vi "pmu_Phasor Scale CFG-3.vi"(8 "phasors in":csg[](array[numeric]), 9 "phasor angle offsets [rad]":sgl[](array[numeric]), 10 "phasor scale factors":sgl[](array[numeric]), 11 "format":u16) -> (2 "phasor out of range":bool, 3 "phasor byte array":u8[](array[numeric]))   [LabVIEW 2014, in "NI_EP_PMU.lvlib"]
uses:
  <vilib>/addons/Electrical Power/PMU/NI_EP_PMU.lvlib
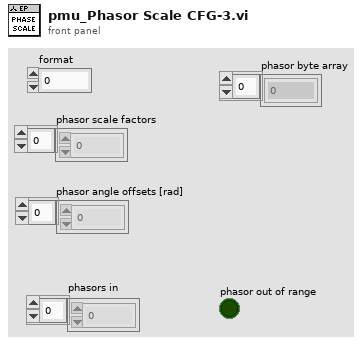
[diagram p1: front panel]
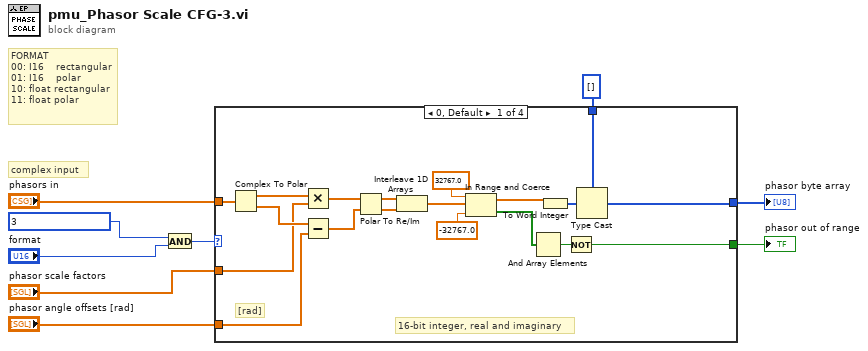
[diagram p0: block diagram]
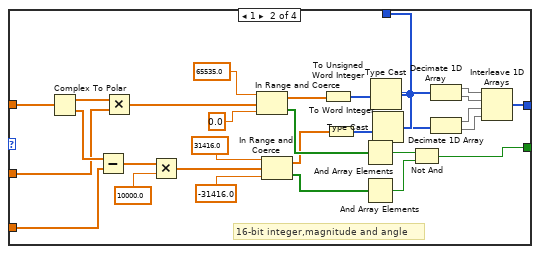
[diagram p2: hidden frame]
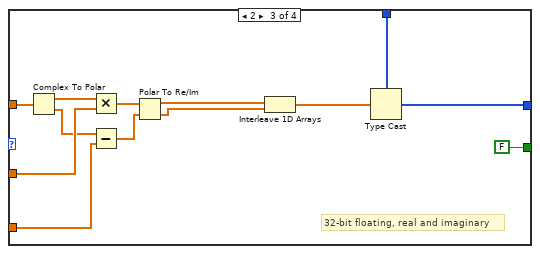
[diagram p3: hidden frame]
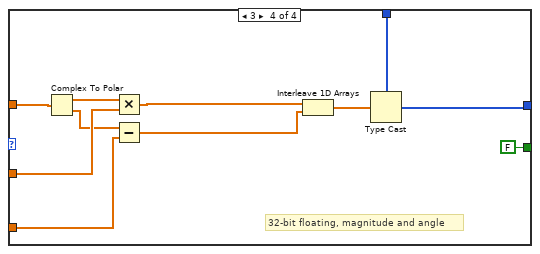
[diagram p4: hidden frame]
diagram:
  # "FORMAT\n00: I16    rectangular\n01: I16    polar\n10: float rectangular\n11: float polar"
  # "complex input"
  n1 = And(x=u16 3, y="format") -> (x .and. y?=w7:u16)
  n2 = case shown="0, Default" w7 {
    tunnel: "phasors in" -> [w23 w58 w67 w78]
    tunnel: u8[] [] ("appended array") -> [w24 w43 w70 w81]
    tunnel: [w28 w36 w69 w80] -> w4
    tunnel: [w25 w35 FALSE FALSE] -> w3
    tunnel: "phasor scale factors" -> [w12 w30 w65 w76]
    tunnel: "phasor angle offsets [rad]" -> [w11 w29 w63 w74]
    frame 0, Default {
      # "[rad]"
      # "16-bit integer, real and imaginary"
      n3 = Complex To Polar(r * e^(i*theta)=w23) -> (r=w22:sgl[], theta=w21:sgl[])
      n4 = Multiply(x=w22, y=w12) -> (x*y=w20:sgl[])
      n5 = Subtract(x=w21, y=w11) -> (x-y=w10:sgl[])
      n6 = Polar To Re/Im(2:w10, 3:w20) -> (0:w18:sgl[], 1:w19:sgl[])
      n7 = Interleave 1D Arrays(w19, w18) -> (w15:sgl[])
      n8 = In Range and Coerce(upper limit=sgl 32767.0, x=w15, lower limit=sgl -32767.0) -> (coerced(x)=w14:sgl[], In Range?=w13:bool[])
      n9 = And Array Elements(Boolean array=w13) -> (logical AND=w26:bool)
      n10 = To Word Integer(number=w14) -> (16bit integer=w27:i16[])
      n11 = Not(x=w26) -> (.not. x?=w25:bool)
      n12 = Type Cast(type=w24, x=w27) -> (*(type *) &x=w28:u8[])
    }
    frame 1 {
      # "16-bit integer,magnitude and angle"
      n13 = Complex To Polar(r * e^(i*theta)=w58) -> (r=w57:sgl[], theta=w34:sgl[])
      n14 = Subtract(x=w34, y=w29) -> (x-y=w32:sgl[])
      n15 = Multiply(x=w57, y=w30) -> (x*y=w56:sgl[])
      n16 = Multiply(x=w32, y=sgl 10000.0) -> (x*y=w33:sgl[])
      n17 = In Range and Coerce(upper limit=sgl 65535.0, x=w56, lower limit=sgl 0.0) -> (coerced(x)=w48:sgl[], In Range?=w51:bool[])
      n18 = In Range and Coerce(upper limit=sgl 31416.0, x=w33, lower limit=sgl -31416.0) -> (coerced(x)=w47:sgl[], In Range?=w45:bool[])
      n19 = To Unsigned Word Integer(number=w48) -> (unsigned 16bit integer=w46:u16[])
      n20 = To Word Integer(number=w47) -> (16bit integer=w44:i16[])
      n21 = And Array Elements(Boolean array=w51) -> (logical AND=w50:bool)
      n22 = And Array Elements(Boolean array=w45) -> (logical AND=w49:bool)
      n23 = Type Cast(type=w43, x=w46) -> (*(type *) &x=w42:u8[])
      n24 = Type Cast(type=w43, x=w44) -> (*(type *) &x=w41:u8[])
      n25 = Not And(1:w49, 2:w50) -> (0:w35:bool)
      n26 = Decimate 1D Array(w42) -> (w40:u8[], w39:u8[])
      n27 = Decimate 1D Array(w41) -> (w38:u8[], w37:u8[])
      n28 = Interleave 1D Arrays(w40, w39, w38, w37) -> (w36:u8[])
    }
    frame 2 {
      # "32-bit floating, real and imaginary"
      n29 = Complex To Polar(r * e^(i*theta)=w67) -> (r=w66:sgl[], theta=w64:sgl[])
      n30 = Multiply(x=w66, y=w65) -> (x*y=w62:sgl[])
      n31 = Subtract(x=w64, y=w63) -> (x-y=w61:sgl[])
      n32 = Polar To Re/Im(2:w61, 3:w62) -> (0:w59:sgl[], 1:w60:sgl[])
      n33 = Interleave 1D Arrays(w60, w59) -> (w71:sgl[])
      n34 = Type Cast(type=w70, x=w71) -> (*(type *) &x=w69:u8[])
    }
    frame 3 {
      # "32-bit floating, magnitude and angle"
      n35 = Complex To Polar(r * e^(i*theta)=w78) -> (r=w77:sgl[], theta=w75:sgl[])
      n36 = Multiply(x=w77, y=w76) -> (x*y=w73:sgl[])
      n37 = Subtract(x=w75, y=w74) -> (x-y=w72:sgl[])
      n38 = Interleave 1D Arrays(w73, w72) -> (w82:sgl[])
      n39 = Type Cast(type=w81, x=w82) -> (*(type *) &x=w80:u8[])
    }
  }
  "phasor byte array" <- w4
  "phasor out of range" <- w3
